vi "U32ArrayToU8Array.vi"(1 "U32-bit Array":u32[](array[numeric])) -> (0 "U8-bit Array":u8[](array[numeric]))   [LabVIEW 2011]
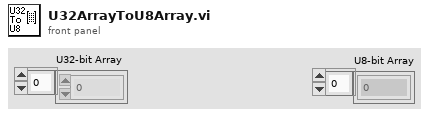
[diagram p1: front panel]
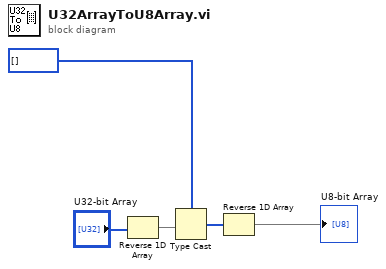
[diagram p0: block diagram]
diagram:
  n1 = Reverse 1D Array(array="U32-bit Array") -> (reversed array=w5:u32[])
  n2 = Type Cast(type=u8[] [], x=w5) -> (*(type *) &x=w2:u8[])
  n3 = Reverse 1D Array(array=w2) -> (reversed array=→"U8-bit Array":u8[])
